vi "SerialPort.Disconnect.vi"(8 "error in (no error)":errorcluster, 11 "SerialPort in":refnum<class "SerialPort.lvclass">) -> (0 "error out":errorcluster, 2 "State":T1, 3 "SerialPort out":refnum<class "SerialPort.lvclass">)   [LabVIEW 2018, in "SerialPort.lvclass"]
uses:
  SerialPort.lvclass
  Controls/SerialPort.Status Enum.ctl
  SerialPort.lvclass/SerialPort.ctl
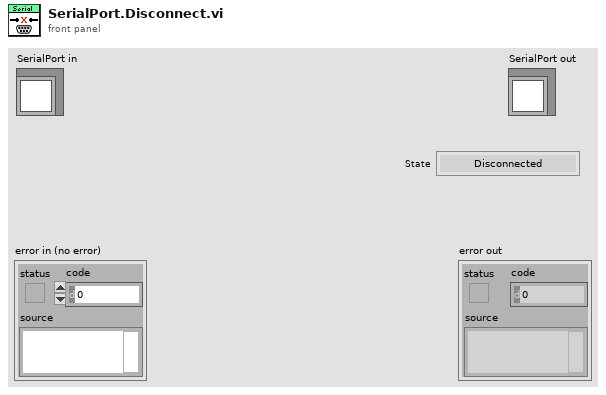
[diagram p1: front panel]
types:
  T1 = typedef "SerialPort.Status Enum.ctl" = enum16{"Disconnected", "Connecting", "Connected"}
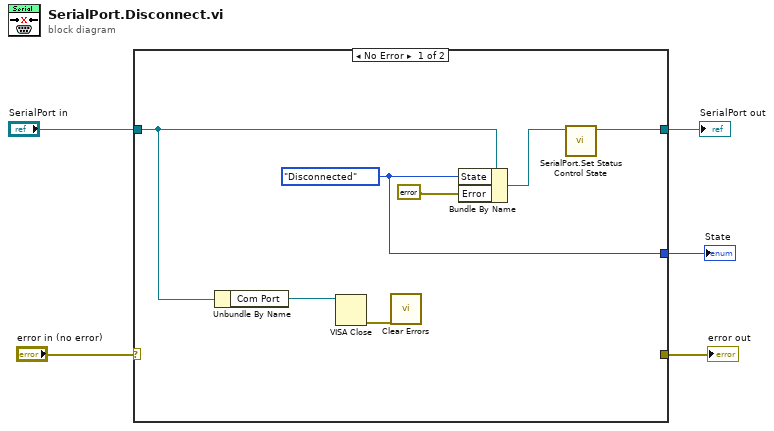
[diagram p0: block diagram]
diagram:
  n1 = case shown="No Error" "error in (no error)" {
    selector: "error in (no error)" -> [_ w14]
    tunnel: [_ w14] -> w4
    tunnel: [w12 w13] -> w2
    tunnel: "SerialPort in" -> [w8 w13]
    tunnel: [w10 _] -> w1
    frame No Error {
      w10 = SerialPort.Status_Enum."Disconnected" ("State")
      n2 = Unbundle By Name(w8) -> ("Com Port"=w7:refnum<visa-resource-name>)
      n3 = VISA Close(VISA resource name=w7) -> (error out=w6:errorcluster)  [unwired: 1 in]
      n4 = call <vilib>:"Clear Errors.vi"("error in (no error)"=w6) -> ()  [unwired: 5 in, 2 out]
      n5 = Bundle By Name(cluster=w8, "State"=w10, "Error"=errorcluster {"status"=FALSE, "code"=0, "source"=""}) -> (w11:refnum<class "SerialPort.lvclass">)
      n6 = call "SerialPort.Set Status Control State.vi"("SerialPort in"=w11) -> ("SerialPort out"=w12:refnum<class "SerialPort.lvclass">)  [unwired: 9 in, 1 out]
    }
    frame Error {
    }
  }
  "error out" <- w4
  "SerialPort out" <- w2
  "State" <- w1
